vi "Scan Engine Init RemIO Mod.vi"(8 "error in (no error)":errorcluster, 10 "SubPanel Ref":refnum<vi>, 11 "Node Ptr In":T1 format="%.0x") -> (0 "error out":errorcluster, 3 "Node Ptr Out":T1 format="%.0x", 5 "SubPanel Command":refnum<user-event>)   [LabVIEW 2019, in "SEECD System Explorer.lvlib"]
uses:
  SEECD System Explorer.lvlib
  <vilib>/NI VeriStand/Custom Device API/Custom Device Item Ref.ctl
  Modules.lvlibp/RSI Module/SubPanel Command.ctl
  Modules.lvlibp/RemIO Module/RemIO Module.lvclass
  Modules.lvlibp/RSI Module/RSI Module.lvclass
  <vilib>/NI VeriStand/Custom Device API/Custom Device API.lvlib
panel:
  out "RemIO Module":refnum<class "RemIO Module.lvclass">
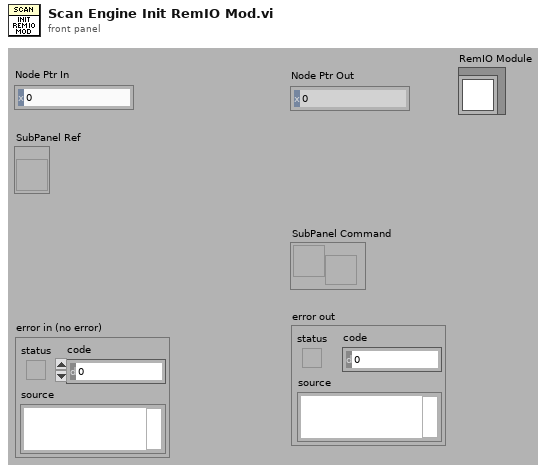
[diagram p1: front panel]
types:
  T1 = typedef "Custom Device API.lvlib/Custom Device Item Ref.ctl" = u64
  T2 = typedef "Modules.lvlibp/RSI Module.lvclass/SubPanel Command.ctl" = enum16{"Stop"}
  T3 = typedef "Modules.lvlibp/Custom Device API.lvlib/Custom Device Item Ref.ctl" = u64
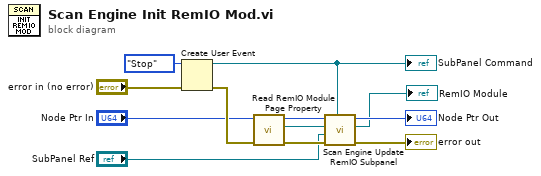
[diagram p0: block diagram]
diagram:
  n1 = Create User Event(user event datatype=SubPanel_Command."Stop" ("SubPanel Command"), error in="error in (no error)") -> (user event=w2:refnum<user-event>, error out=w10:errorcluster)
  "SubPanel Command" <- w2
  n2 = call "Read RemIO Module Page Property.vi"("error in (no error)"=w10, "Node Ptr In"="Node Ptr In") -> ("error out"=w8:errorcluster, "RemIO Module"=w4:refnum<class "RemIO Module.lvclass">, "Node Ptr Out"=w3:T3)  [unwired: 7 in]
  n3 = call "Scan Engine Update RemIO Subpanel.vi"("SubPanel Event"=w2, "error in (no error)"=w8, "SubPanel Ref"="SubPanel Ref", "RemIO Module In"=w4, "Node Ptr In"=w3) -> ("error out"=→"error out":errorcluster, "RemIO Module Out"=→"RemIO Module":refnum<class "RemIO Module.lvclass">, "Node Ptr Out"=→"Node Ptr Out":T1)  [unwired: 4 in]
